vi "Get_ACIR_Test_Data2.vi"(8 "error in (no error)":errorcluster caption="错误输入（无错误）", 11 "VISA引用句柄输入":refnum<visa-resource-name>) -> (0 "error out":errorcluster caption="错误输出", 1 "读取缓冲区":string, 2 "读取缓冲区 2":string, 3 "VISA引用句柄输出":refnum<visa-resource-name>)   [LabVIEW 2018]
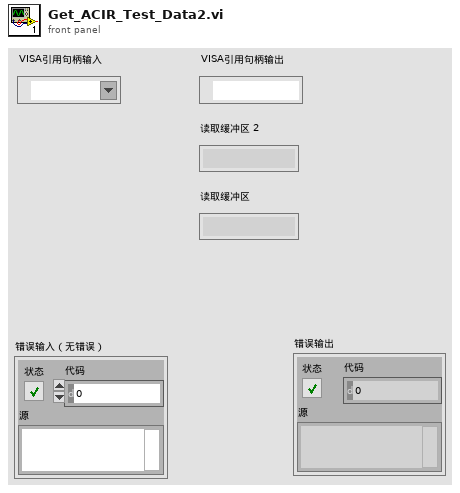
[diagram p1: front panel]
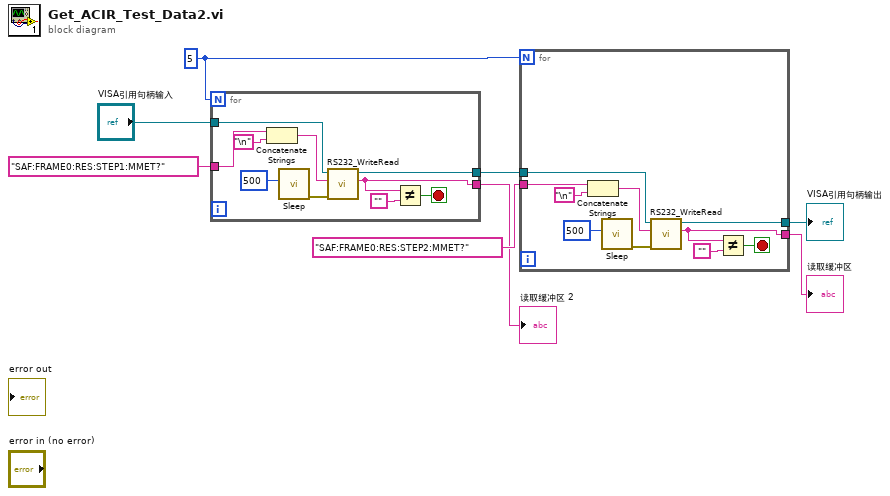
[diagram p0: block diagram]
diagram:
  w7 = 5
  n1 = for {
    N: w7 -> [_]
    tunnel: "SAF:FRAME0:RES:STEP1:MMET?" ("写入缓冲区") -> [w18]
    tunnel: [w10] -> w3
    tunnel: "VISA引用句柄输入" -> [w15]
    tunnel: [w14] -> w5
    stop <- w9 stop-if-true
    n2 = Concatenate Strings(w18, "\n") -> (w16:string)
    n3 = call "Sleep.vi"("等待时间（毫秒）"=u32 500) -> ("error out"=w12:errorcluster)  [unwired: 10 in]
    n4 = call "RS232_WriteRead.vi"("错误输入（无错误）"=w12, "写入缓冲区"=w16, "VISA资源名称"=w15) -> ("读取缓冲区"=w10:string, "VISA资源名称输出"=w14:refnum<visa-resource-name>)  [unwired: 6 in, 1 out]
    n5 = Not Equal?(x=w10, y="") -> (x != y?=w9:bool)
  }
  "读取缓冲区 2" <- w3
  n6 = for {
    N: w7 -> [_]
    tunnel: "SAF:FRAME0:RES:STEP2:MMET?" ("写入缓冲区") -> [w28]
    tunnel: [w20] -> w8
    tunnel: w5 -> [w25]
    tunnel: [w24] -> w6
    stop <- w19 stop-if-true
    n7 = Concatenate Strings(w28, "\n") -> (w26:string)
    n8 = call "Sleep.vi"("等待时间（毫秒）"=u32 500) -> ("error out"=w22:errorcluster)  [unwired: 10 in]
    n9 = call "RS232_WriteRead.vi"("错误输入（无错误）"=w22, "写入缓冲区"=w26, "VISA资源名称"=w25) -> ("读取缓冲区"=w20:string, "VISA资源名称输出"=w24:refnum<visa-resource-name>)  [unwired: 6 in, 1 out]
    n10 = Not Equal?(x=w20, y="") -> (x != y?=w19:bool)
  }
  "读取缓冲区" <- w8
  "VISA引用句柄输出" <- w6
